vi "run.vi"(8 "error in (no error)":errorcluster, 11 "CommandProcessor in":refnum<class "CommandProcessor.lvclass">) -> (0 "error out":errorcluster, 3 "CommandProcessor out":refnum<class "CommandProcessor.lvclass">)   [LabVIEW 2009, in "Tools.lvlib" / "Interpreters.lvlib" / "CommandProcessor.lvclass"]
uses:
  CommandProcessor.lvclass
  CommandProcessor.lvclass/CommandProcessor.ctl
  SettingsEventManager/SettingsEventsManager.lvclass
  CommandEvents/CommandEvents.lvclass
panel:
  in  "commandKey":T1(ring)
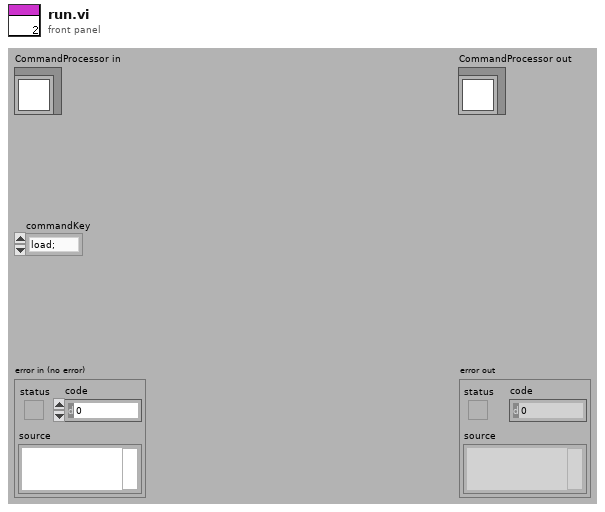
[diagram p1: front panel]
types:
  T1 = enum16{"load;", "lookup;", "replace;", "save;", "close;", "use;", "nodePath;", "valuePath;", "?;", "info;", "insertNode;"}
  T2 = cluster{"newCommand":refnum<user-event>, "textUpdate":refnum<user-event>}
  T3 = cluster{"settingsFrontEndEvents":cluster{"loadSettingsFromPath":refnum<user-event>, "lookUpElementEvent":refnum<user-event>, "saveSettings":refnum<user-event>, "loadSettings":refnum<user-event>, "close":refnum<user-event>, "replaceElement":refnum<user-event>, "findParentNodes":refnum<user-event>, "createNode":refnum<user-event>}, "settingBackEndEvents":cluster{"defaultSettingsPathRequest":refnum<user-event>, "searchResultEvent":refnum<user-event>, "settingsSaved":refnum<user-event>, "settingsLoaded":refnum<user-event>, "foundParentNode":refnum<user-event>}}
  T4 = cluster{"loadSettingsFromPath":refnum<user-event>, "lookUpElementEvent":refnum<user-event>, "saveSettings":refnum<user-event>, "loadSettings":refnum<user-event>, "close":refnum<user-event>, "replaceElement":refnum<user-event>, "findParentNodes":refnum<user-event>, "createNode":refnum<user-event>}
  T5 = cluster{"defaultSettingsPathRequest":refnum<user-event>, "searchResultEvent":refnum<user-event>, "settingsSaved":refnum<user-event>, "settingsLoaded":refnum<user-event>, "foundParentNode":refnum<user-event>}
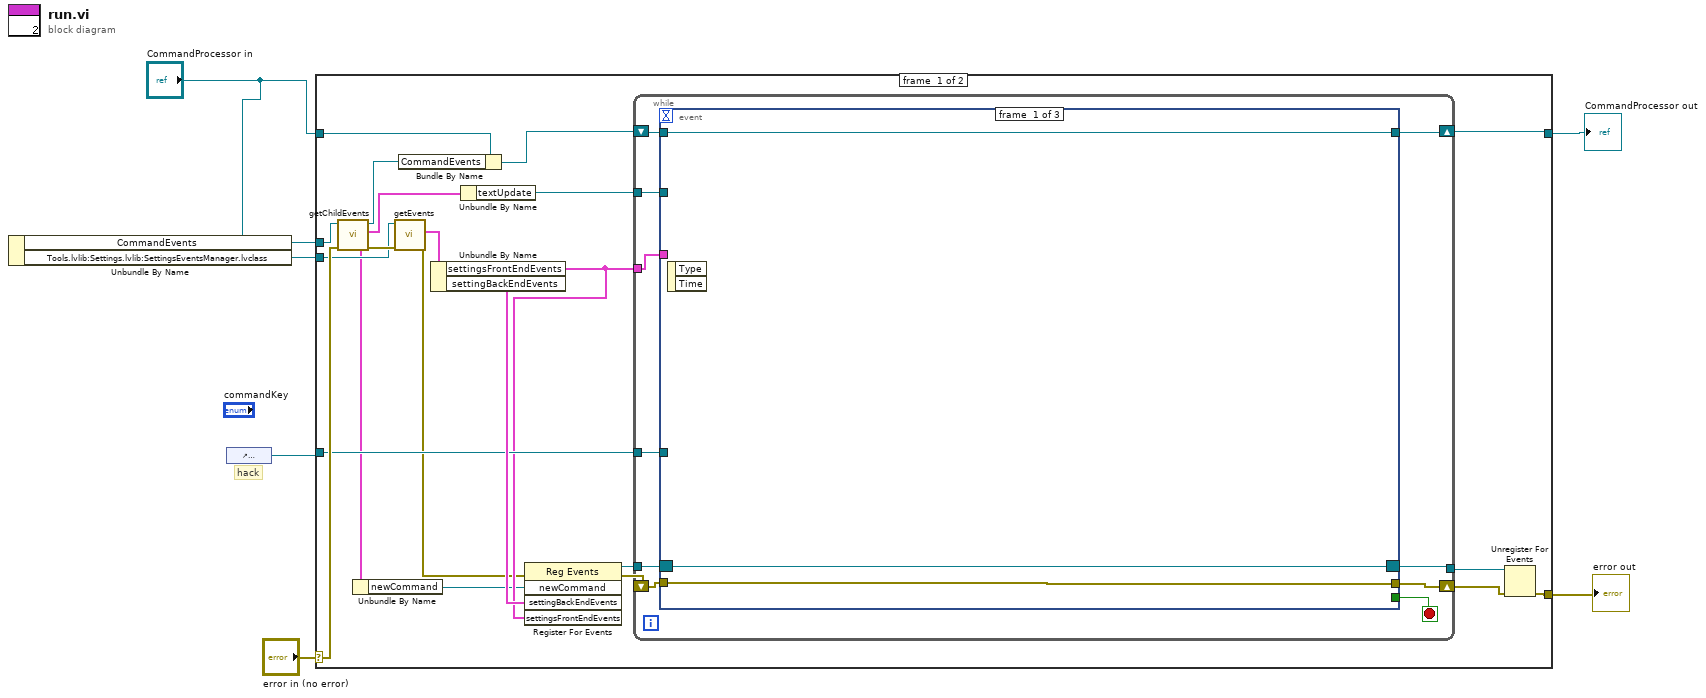
[diagram p0: block diagram]
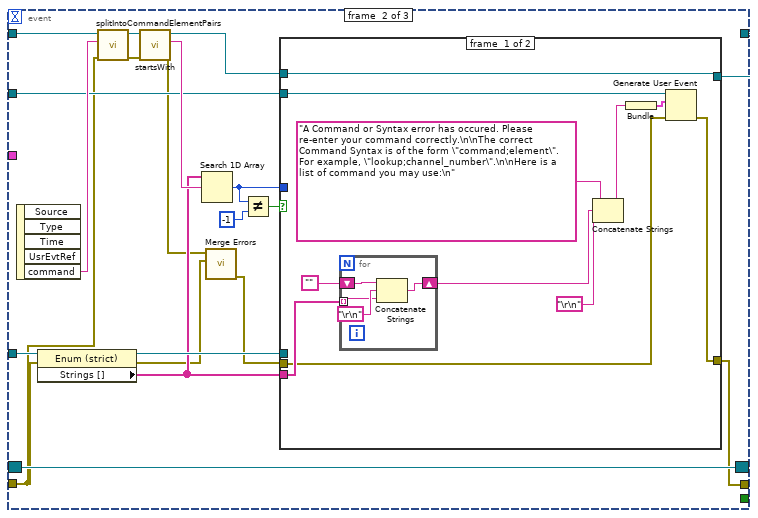
[diagram p2: hidden frame]
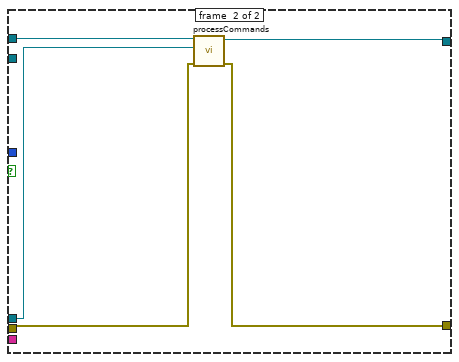
[diagram p3: hidden frame]
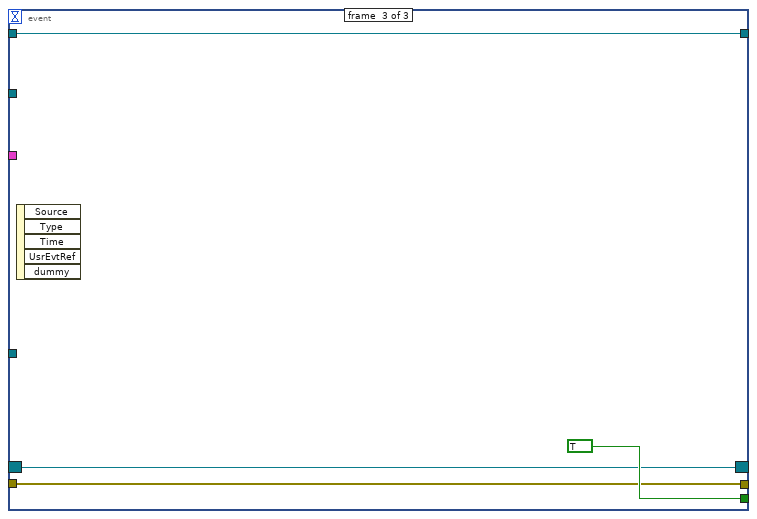
[diagram p4: hidden frame]
diagram:
  # "hack"
  n1 = Unbundle By Name("CommandProcessor in") -> ("CommandEvents"=w2:refnum<class "CommandEvents.lvclass">, "Tools.lvlib:Settings.lvlib:SettingsEventsManager.lvclass"=w3:refnum<class "SettingsEventsManager.lvclass">)
  n2 = control-ref of="commandKey"() -> (w1:refnum<vi>)
  n3 = case shown="No Error" "error in (no error)" {
    selector: "error in (no error)" -> [w22 w87]
    tunnel: [w23 w87] -> w7
    tunnel: [w28 w86] -> w6
    tunnel: "CommandProcessor in" -> [w17 w86]
    tunnel: w1 -> [w19 _]
    tunnel: w3 -> [w11 _]
    tunnel: w2 -> [w10 _]
    frame #0 {
      n4 = call-dynamic "getChildEvents.vi"("error in (no error)"=w22, "CommandEvents in"=w10) -> ("error out"=w15:errorcluster, "Events"=w9:T2, "CommandEvents out"=w14:refnum<class "CommandEvents.lvclass">)  [unwired: 7 in]
      n5 = Unbundle By Name(w9) -> ("newCommand"=w8:refnum<user-event>)
      n6 = call-dynamic "getEvents.vi"("error in (no error)"=w15, "SettingsEventsManager in"=w11) -> ("error out"=w12:errorcluster, "settingsEvents"=w13:T3)  [unwired: 7 in, 1 out]
      n7 = Bundle By Name(cluster=w17, "CommandEvents"=w14) -> (w16:refnum<class "CommandProcessor.lvclass">)
      n8 = Unbundle By Name(w13) -> ("settingsFrontEndEvents"=w18:T4, "settingBackEndEvents"=w21:T5)
      n9 = Unbundle By Name(w9) -> ("textUpdate"=w20:refnum<user-event>)
      n10 = register-events(error in=w12, w8, w21, w18) -> (reference out=w27:refnum<event-registration>, error out=w26:errorcluster)  [unwired: 1 in]
      n11 = while {
        shift-right: [w35] -> w24
        shift-left: w26 -> [w36]
        shift-right: [w37] -> w28
        shift-left: w16 -> [w38]
        tunnel: w27 -> [w34]
        tunnel: [w33] -> w25
        tunnel: w18 -> [w32]
        tunnel: w20 -> [w31]
        tunnel: w19 -> [w30]
        stop <- w29 stop-if-true
        n12 = event shown="[1] <newCommand>: User Event" {
          selector: w34 -> [w40 w61 w83]
          dyn-events: [w40 w61 w83] -> w33
          timeout: _ -> [_ _ _]
          tunnel: w38 -> [w39 w60 w82]
          tunnel: [w39 w42 w82] -> w37
          tunnel: w36 -> [w41 w47 w84]
          tunnel: [w41 w50 w84] -> w35
          tunnel: w32 -> [_ _ _]
          tunnel: w31 -> [_ w49 _]
          tunnel: w30 -> [_ w56 _]
          tunnel: [_ _ TRUE] -> w29
          event #0 {
            n13 = event-data() -> ()  [unwired: 1 in, 2 out]
          }
          event #1 {
            n14 = event-data() -> ("command"=w59:string)  [unwired: 1 in, 4 out]
            n15 = property class="Enum (strict)"(reference=w56, error in=w47) -> (reference out=w52:refnum<vi>, error out=w45:errorcluster, "Strings []"=w48:string[])
            n16 = call-dynamic "splitIntoCommandElementPairs.vi"("error in (no error)"=w47, "command"=w59, "CommandProcessor in"=w60) -> ("error out"=w58:errorcluster, "CommandProcessor out"=w57:refnum<class "CommandProcessor.lvclass">)  [unwired: 7 in]
            n17 = call-dynamic "startsWith.vi"("error in (no error)"=w58, "CommandProcessor in"=w57) -> ("error out"=w46:errorcluster, "command"=w55:string, "CommandProcessor out"=w43:refnum<class "CommandProcessor.lvclass">)  [unwired: 6 in, 1 out]
            n18 = Search 1D Array(1D array=w48, element=w55) -> (index of element=w51:i32)  [unwired: 1 in]
            n19 = call <vilib>:"Merge Errors.vi"("error in 2 (no error)"=w45, "error in 1 (no error)"=w46) -> ("error out"=w44:errorcluster)  [unwired: 5 in]
            n20 = Not Equal?(x=w51, y=-1) -> (x != y?=w53:bool)
            n21 = case shown="True" w53 {
              tunnel: w52 -> [_ w77]
              tunnel: w51 -> [_ _]
              tunnel: w44 -> [w64 w79]
              tunnel: [w63 w78] -> w50
              tunnel: w49 -> [w72 _]
              tunnel: w48 -> [w71 _]
              tunnel: w43 -> [w62 w81]
              tunnel: [w62 w80] -> w42
              frame #0 {
                n22 = for {
                  tunnel: w71 -> [w74] mode=indexing
                  shift-right: [w73] -> w68
                  shift-left: "" -> [w76]
                  n23 = Concatenate Strings(w76, "\r\n", w74) -> (w73:string)
                }
                n24 = Concatenate Strings("A Command or Syntax error has occured. Please re-enter your command correctly.\n\nThe correct Command Syntax is of the form \"command;element\". For example, \"lookup;channel_number\".\n\nHere is a list of command you may use:\n", w68, "\r\n") -> (w66:string)
                n25 = Bundle(w66) -> (w65:cluster{string})  [unwired: 1 in]
                n26 = Generate User Event(user event=w72, event data cluster=w65, error in=w64) -> (error out=w63:errorcluster)  [unwired: 1 out]
              }
              frame #1 {
                n27 = call-dynamic "processCommands.vi"("error in (no error)"=w79, "commandKey"=w77, "CommandProcessor in"=w81) -> ("error out"=w78:errorcluster, "CommandProcessor out"=w80:refnum<class "CommandProcessor.lvclass">)  [unwired: 7 in]
              }
            }
          }
          event #2 {
            n28 = event-data() -> ()  [unwired: 1 in, 5 out]
          }
        }
      }
      n29 = Unregister For Events(event registration refnum=w25, error in=w24) -> (error out=w23:errorcluster)
    }
    frame #1 {
    }
  }
  "error out" <- w7
  "CommandProcessor out" <- w6
